vi "Example Auto Hold Mode.vi"() -> ()   [LabVIEW 2021]
doc: "This VI exampe shows how to use the Auto hold mode of the instrument U1282A. It uses the Read block of the U1282A library to perform the reading of the measurement."
uses:
  Keysight U1282A.lvlib
panel:
  in  "Trigger Count":dbl=50.0 min=0.0 max=9999.0 step=1.0
  in  "VISA resource name":refnum<visa-resource-name>="Keysight_U1282A"
  out "Reading":dbl
  in  "Read":bool
  in  "Salir":bool
  # "This VI example allows the user to perform measurements using the Auto Hold mode of the instrument U1282A. Use the Trigger Count control to set the count for the trigger of the instrument. The reading of the primary display of the instrument is presented in the Reading indicator when the button Read is pressed."
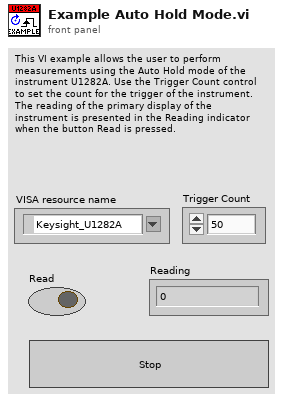
[diagram p1: front panel]
types:
  T1 = cluster{"Baud Rate":enum16{"1200", "2400", "4800", "9600", "19200", "38400", "57600", "115200"}, "Timeout":u32, "Stop Bits":u16, "Flow Control":enum16{"None", "XON / XOFF", "RTS / CTS", "DTR / DSR"}, "Parity":u16}
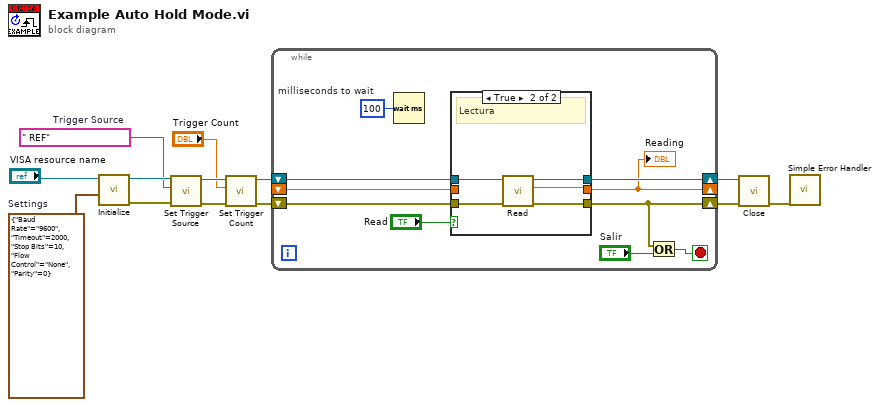
[diagram p0: block diagram]
diagram:
  w8 = T1 {"Baud Rate"=enum."9600", "Timeout"=2000, "Stop Bits"=10, "Flow Control"=enum."None", "Parity"=0}  # Settings
  w9 = " REF"  # Trigger Source
  n1 = call "Initialize.vi"("Settings"=w8, "VISA resource name"="VISA resource name") -> ("error out"=w13:errorcluster, "VISA resource name out"=w12:refnum<visa-resource-name>)  [unwired: 8 in]
  n2 = call "Set Trigger Source.vi"("error in"=w13, "Trigger Source"=w9, "VISA resource name in"=w12) -> ("error out"=w6:errorcluster, "VISA resource name out"=w3:refnum<visa-resource-name>)  [unwired: 7 in]
  n3 = call "Set Trigger Count.vi"("error in"=w6, "Count"="Trigger Count", "VISA resource name in"=w3) -> ("error out"=w5:errorcluster, "VISA resource name out"=w4:refnum<visa-resource-name>)  [unwired: 7 in]
  n4 = while {
    shift-right: [w16] -> w11
    shift-left: w5 -> [w21]
    shift-right: [w22] -> w10
    shift-left: w4 -> [w20]
    shift-right: [w18] -> _
    shift-left: _ -> [w19]
    stop <- w15 stop-if-true
    w14 = u32 100  # milliseconds to wait
    n5 = Wait (ms)(milliseconds to wait=w14) -> ()  [unwired: 1 out]
    n6 = case shown="True" "Read" {
      tunnel: [w25 w30] -> w16
      tunnel: [w24 w27] -> w18
      tunnel: [w26 w28] -> w22
      tunnel: w21 -> [w25 w31]
      tunnel: w20 -> [w26 w29]
      tunnel: w19 -> [w24 _]
      frame False {
      }
      frame True {
        # "Lectura"
        n7 = call "Read.vi"("error in"=w31, "VISA resource name in"=w29) -> ("error out"=w30:errorcluster, "Value"=w27:dbl, "VISA resource name out"=w28:refnum<visa-resource-name>)  [unwired: 7 in]
      }
    }
    "Reading" <- w18
    n8 = Or(x=w16, y="Salir") -> (x .or. y?=w15:bool)
  }
  n9 = call "Close.vi"("error in"=w11, "VISA resource name"=w10) -> ("error out"=w1:errorcluster)  [unwired: 9 in]
  n10 = call <vilib>:"Simple Error Handler.vi"("error in (no error)"=w1) -> ()  [unwired: 4 in, 5 out]
